vi "update_enum_string_with_cmd_info.vi"(9 "vi path":path=path "C:/Program Files (x86)/National Instruments/LabVIEW 2011/instr.lib/Express/Utility/gen_node.vi", 10 "CmdInfo":T1) -> (2 "CmdInfo Out":T1)   [LabVIEW 2018]
uses:
  command_spec.ctl
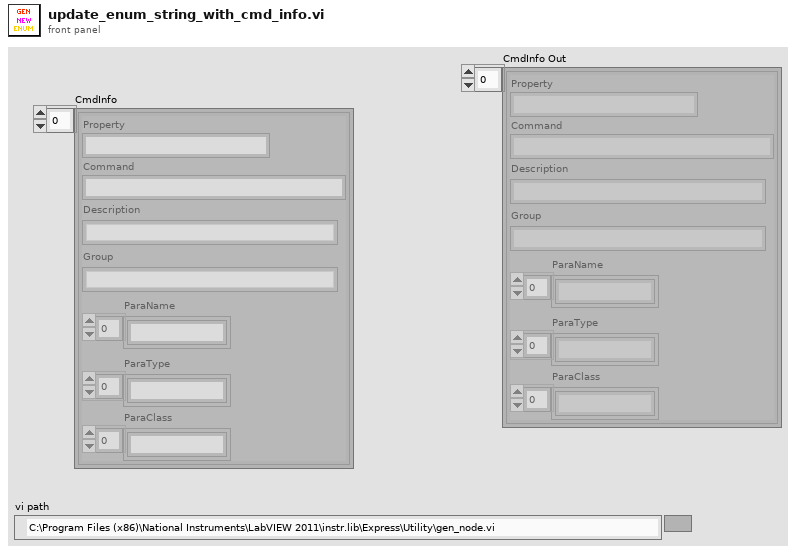
[diagram p1: front panel]
types:
  T1 = typedef "command_spec.ctl" = cluster{"Property":string, "Command":string, "Description":string, "Group":string, "ParaName":string[], "ParaType":string[], "ParaClass":string[]}[]
  T2 = typedef "auto_extracted_control_specs.ctl" = T3[]
  T3 = typedef "auto_extracted_control_spec.ctl" = cluster{"Control Data Type":T4, "Ring Text":string[], "Control Label":string, "Command Start Offset":i32, "Command Stop Offset":i32, "Control Class":T5, "Default Value":string, "Ring Strings and Values":T6[]}
  T4 = typedef "control_data_type.ctl" = enum16{"DBL", "I32", "Boolean", "String", "U16", "U32", "EXT", "SGL", "I16", "U8", "I8", "I64", "U64", "Waveform", "Reference", "Variant", "Cluster"}
  T5 = typedef "control_class.ctl" = enum16{"Numeric", "Vertical Slide Switch", "Text Ring", "String", "Array", "VISAName", "WaveformGraph", "Cluster"}
  T6 = typedef "ring_string_and_value.ctl" = cluster{"String":string, "Value":dbl}
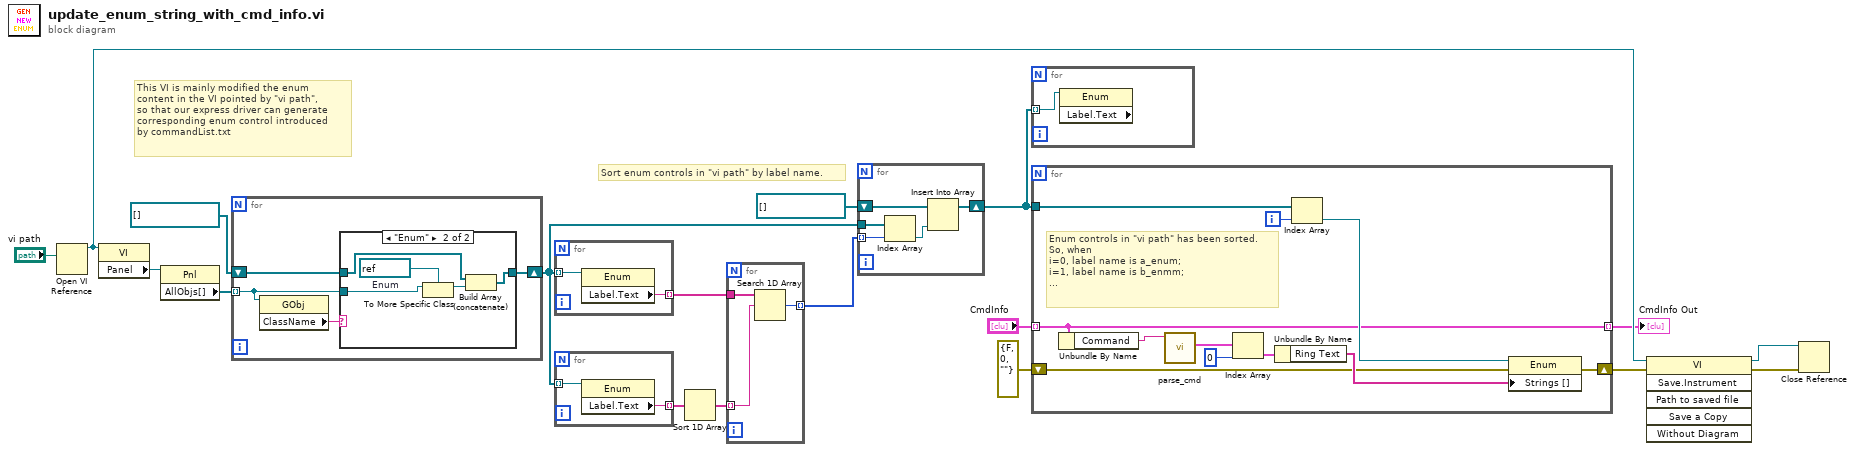
[diagram p0: block diagram]
diagram:
  # "Sort enum controls in \"vi path\" by label name."
  # "This VI is mainly modified the enum\ncontent in the VI pointed by \"vi path\",\nso that our express driver can generate\ncorresponding enum control introduced\nby commandList.txt"
  n1 = Open VI Reference(vi path="vi path") -> (vi reference=w9:refnum<vi>)  [unwired: 5 in, 1 out]
  n2 = property class="VI"(reference=w9) -> ("Panel"=w18:refnum<vi>)  [unwired: 1 in, 2 out]
  n3 = property class="Pnl"(reference=w18) -> ("AllObjs[]"=w1:refnum<vi>[])  [unwired: 1 in, 2 out]
  n4 = for {
    tunnel: w1 -> [w22] mode=indexing
    shift-right: [w20] -> w12
    shift-left: refnum<vi>[] [] -> [w21]
    n5 = property class="GObj"(reference=w22) -> ("ClassName"=w19:string)  [unwired: 1 in, 2 out]
    n6 = case shown="\"Enum\"" w19 {
      tunnel: w22 -> [_ w27]
      tunnel: w21 -> [w23 w24]
      tunnel: [w23 w25] -> w20
      frame "False", Default {
      }
      frame "Enum" {
        w28 = refnum<vi> refnum  # Enum
        n7 = To More Specific Class(target class=w28, reference=w27) -> (specific class reference=w26:refnum<vi>)  [unwired: 1 in, 1 out]
        n8 = Build Array (concatenate)(w24, w26) -> (w25:refnum<vi>[])
      }
    }
  }
  n9 = for {
    tunnel: w12 -> [w30] mode=indexing
    tunnel: [w29] -> w14 mode=indexing
    n10 = property class="Enum"(reference=w30) -> ("Label.Text"=w29:string)  [unwired: 1 in, 2 out]
  }
  n11 = for {
    tunnel: w12 -> [w32] mode=indexing
    tunnel: [w31] -> w15 mode=indexing
    n12 = property class="Enum"(reference=w32) -> ("Label.Text"=w31:string)  [unwired: 1 in, 2 out]
  }
  n13 = Sort 1D Array(array=w15) -> (sorted array=w10:string[])
  n14 = for {
    tunnel: w14 -> [w35]
    tunnel: w10 -> [w34] mode=indexing
    tunnel: [w33] -> w13 mode=indexing
    n15 = Search 1D Array(1D array=w35, element=w34) -> (index of element=w33:i32)  [unwired: 1 in]
  }
  n16 = for {
    tunnel: w13 -> [w39] mode=indexing
    tunnel: w12 -> [w40]
    shift-right: [w37] -> w8
    shift-left: refnum<vi>[] [] -> [w36]
    n17 = Index Array(array=w40, index=w39) -> (element=w38:refnum<vi>)
    n18 = Insert Into Array(array=w36, new element=w38) -> (w37:refnum<vi>[])  [unwired: 1 in]
  }
  n19 = for {
    tunnel: w8 -> [w41] mode=indexing
    n20 = property class="Enum" props=["Label", "Text"](reference=w41) -> ()  [unwired: 1 in, 3 out]
  }
  n21 = for {
    tunnel: "CmdInfo" -> [w42] mode=indexing
    tunnel: w8 -> [w46]
    shift-right: [w44] -> w7
    shift-left: errorcluster {"status"=FALSE, "code"=0, "source"=""} ("error out") -> [w43]
    tunnel: [w42] -> w6 mode=indexing
    i -> [w47]
    # "Enum controls in \"vi path\" has been sorted.\nSo, when \ni=0, label name is a_enum; \ni=1, label name is b_enmm;\n..."
    n22 = Unbundle By Name(w42) -> ("Command"=w52:string)
    n23 = call "parse_cmd.vi"("CMD In"=w52) -> ("CMD Parameters"=w51:T2)  [unwired: 6 in, 4 out]
    n24 = Index Array(array=w51, index=0) -> (element=w49:T3)
    n25 = Unbundle By Name(w49) -> ("Ring Text"=w48:string[])
    n26 = Index Array(array=w46, index=w47) -> (element=w45:refnum<vi>)
    n27 = property class="Enum"(reference=w45, error in=w43, "Strings []"=w48) -> (error out=w44:errorcluster)  [unwired: 1 out]
  }
  "CmdInfo Out" <- w6
  n28 = invoke class="VI" method="Save.Instrument"(reference=w9, error in=w7) -> (reference out=w5:refnum<vi>, error out=w4:errorcluster)  [unwired: 4 in, 4 out]
  n29 = Close Reference(reference=w5, error in (no error)=w4) -> ()  [unwired: 1 out]
